vi "emptyLoop.vi"() -> ()   [LabVIEW 2012]
panel:
  out "Numeric":dbl
  in  "stop":bool
  # "This empty, non-terminating loop can be used to test whether the system can run Labview VIs\nat the same time as Coulbourn Graphic State RT, which is also LV based"
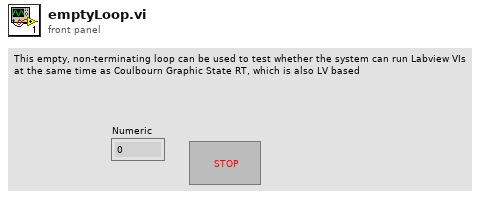
[diagram p1: front panel]
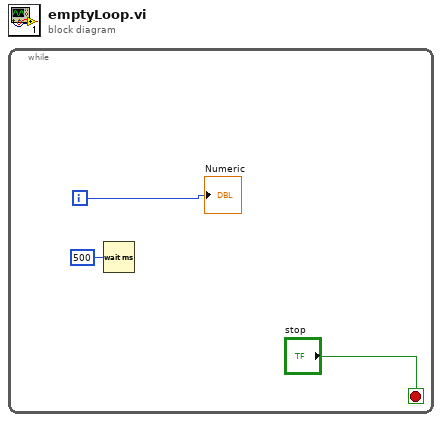
[diagram p0: block diagram]
diagram:
  n1 = while {
    i -> [w2]
    stop <- "stop" stop-if-true
    n2 = Wait (ms)(milliseconds to wait=u32 500) -> ()  [unwired: 1 out]
    "Numeric" <- w2
  }
